vi "Configure Frequency Offset.vi"(0 "VISA resource name":refnum<visa-resource-name>, 5 "Enable Offset (F:Disable)":bool, 7 "Offset Frequency (0Hz)":dbl min=-100.0 max=100000000000.0, 11 "error in (no error)":errorcluster) -> (4 "VISA resource name out":refnum<visa-resource-name>, 15 "error out":errorcluster)   [LabVIEW 2020, in "Anritsu Signal Analyzer Series.lvlib"]
doc: "Configures the frequency offset of the spectrum analyzer."
uses:
  Anritsu Signal Analyzer Series.lvlib
panel:
  # "Hz"
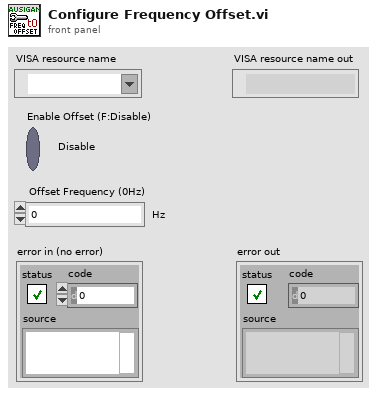
[diagram p1: front panel]
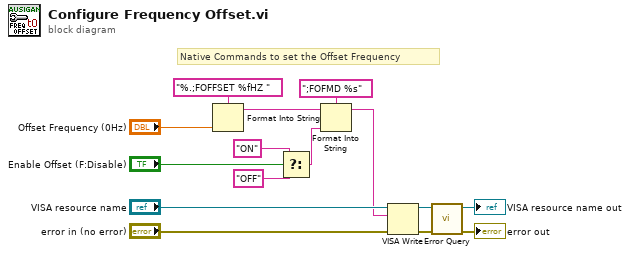
[diagram p0: block diagram]
diagram:
  # "Native Commands to set the Offset Frequency"
  n1 = Format Into String(format string="%.;FOFFSET %fHZ " ("Format String"), "Offset Frequency (0Hz)") -> (resulting string=w6:string)  [unwired: 2 in, 1 out]
  n2 = Select(t="ON" ("複数行文字列"), s="Enable Offset (F:Disable)", f="OFF" ("複数行文字列")) -> (s? t:f=w3:string)
  n3 = Format Into String(format string=";FOFMD %s", initial string=w6, w3) -> (resulting string=w2:string)  [unwired: 1 in, 1 out]
  n4 = VISA Write(VISA resource name="VISA resource name", write buffer=w2, error in (no error)="error in (no error)") -> (VISA resource name out=w8:refnum<visa-resource-name>, error out=w9:errorcluster)  [unwired: 1 out]
  n5 = call "Error Query.vi"("error in (no error)"=w9, "VISA resource name"=w8) -> ("error out"=→"error out":errorcluster, "VISA resource name out"=→"VISA resource name out":refnum<visa-resource-name>)  [unwired: 6 in, 2 out]
